vi "HENES.vi"() -> ()   [LabVIEW 2024]
uses:
  <vilib>/Instr/_visa.llb/VISA Set IO Buffer Mask.ctl
  <vilib>/Instr/_visa.llb/VISA Flush IO Buffer Mask.ctl
  <vilib>/Instr/_visa.llb/VISA Configure Serial Port (Instr).vi
panel:
  in  "탭 컨트롤":enum32{"Main"}(tab)
  in  "HLV_A/M":bool=TRUE
  out "Remote_M/A":bool
  out "E-STOP":bool=TRUE
  out "Alive_PCU":u8(slide)=1 scale=0.0..254.0
  out "Speed_Feed(RPM)":dbl format="%#_g rpm"
  in  "HLV_E-stop":bool
  out "Speed_Feed(m/s)":dbl
  in  "InputSteer(cmd)":dbl=28.559259641865033
  out "Steer_Feed":dbl=-0.28
  in  "HLV_Gear":u8
  out "Gear_Feed":u8=1
  out "HENES Loop Time":u32=48
  in  "HENES":refnum<visa-resource-name>="COM3"
  out "버퍼 읽기":string
  out "버퍼 쓰기":string
  in  "InputSpeed":i16
  in  "stop":bool
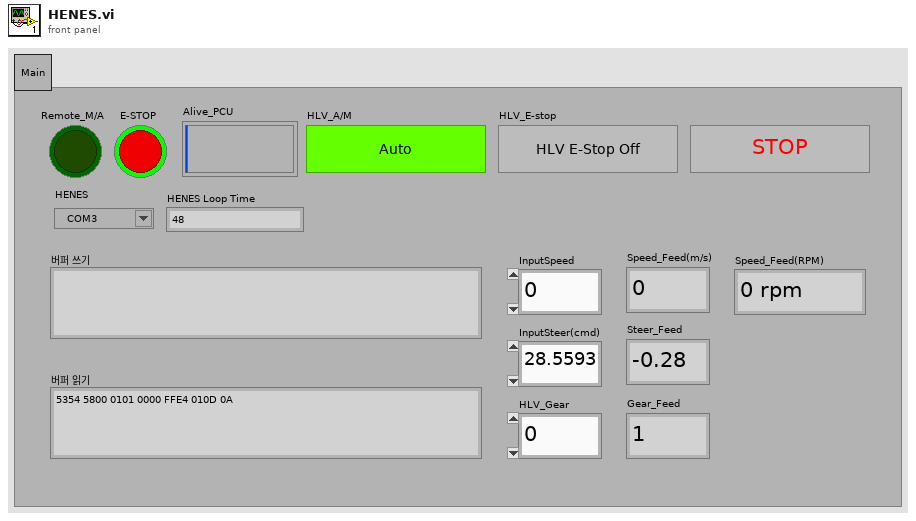
[diagram p1: front panel]
types:
  T1 = cluster{"HENES_M/A":u8, "HENES_E-Stop":u8, "HENES_Gear":u8, "HENES_Speed":i16, "HENES_Steer":i16, "HENES_Alive":u8}
  T2 = typedef "VISA Flush IO Buffer Mask.ctl" = u16
  T3 = typedef "VISA Set IO Buffer Mask.ctl" = u16
  T4 = cluster{"HLV_M/A_Status":u8, "HLV_E-Stop":u8, "HLV_Gear":u8, "HLV_Speed":i16, "HLV_Steer":i16, "HLV_Alive":u8}
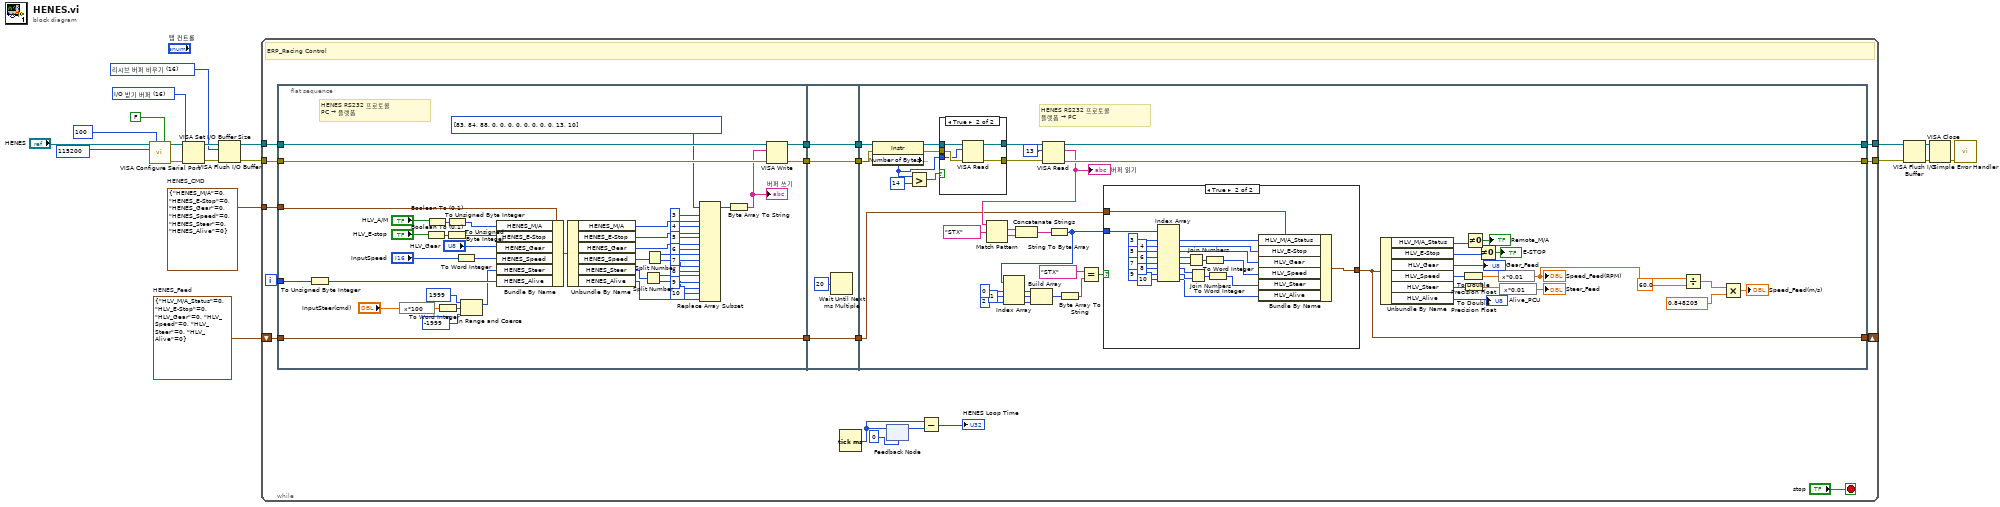
[diagram p0: block diagram]
diagram:
  w2 = T1 {"HENES_M/A"=0, "HENES_E-Stop"=0, "HENES_Gear"=0, "HENES_Speed"=0, "HENES_Steer"=0, "HENES_Alive"=0}  # HENES_CMD
  w5 = T2 16 items=["리시브 버퍼 비우기"=16, "전달 버퍼 디바이스에 쓰기"=32, "리시브 버퍼 비우기(I/O 없음)"=64, "전달 버퍼 비우기"=128] ("Mask")
  w8 = T3 16 items=["I/O 받기 버퍼"=16, "I/O 전달 버퍼"=32, "I/O 받기와 전달 버퍼"=48] ("Mask")
  w12 = T4 {"HLV_M/A_Status"=0, "HLV_E-Stop"=0, "HLV_Gear"=0, "HLV_Speed"=0, "HLV_Steer"=0, "HLV_Alive"=0}  # HENES_Feed
  n1 = call-poly "VISA Configure Serial Port"("VISA resource name"="HENES", "timeout (10sec)"=u32 100, "Enable Termination\nChar (T)"=FALSE ("Enable Termination\nChar (T)"), "baud rate (9600)"=u32 115200) -> ("VISA resource name out"=w4:refnum<visa-resource-name>, "error out"=w3:errorcluster)  [unwired: 10 in]
  n2 = VISA Set I/O Buffer Size(VISA resource name=w4, mask (16)=w8, error in (no error)=w3) -> (VISA resource name out=w7:refnum<visa-resource-name>, error out=w6:errorcluster)  [unwired: 1 in]
  n3 = VISA Flush I/O Buffer(VISA resource name=w7, mask (16)=w5, error in (no error)=w6) -> (VISA resource name out=w17:refnum<visa-resource-name>, error out=w16:errorcluster)
  n4 = while {
    tunnel: w17 -> [w38]
    tunnel: w16 -> [w37]
    tunnel: [w31] -> w15
    tunnel: [w30] -> w14
    shift-right: [w25] -> _
    shift-left: w12 -> [w28]
    tunnel: w2 -> [w26]
    i -> [w32]
    stop <- "stop" stop-if-true
    # "ERP_Racing Control"
    n5 = flat-sequence {
      tunnel: [w81] -> w35
      tunnel: [w80] -> w33
      tunnel: w38 -> [w83]
      tunnel: w37 -> [w82]
      tunnel: w32 -> [w79]
      tunnel: [w78] -> w29
      tunnel: w28 -> [w78]
      tunnel: w26 -> [w77]
      tunnel: [w87] -> w36
      tunnel: w35 -> [w87]
      tunnel: [w86] -> w34
      tunnel: w33 -> [w86]
      tunnel: w29 -> [w84]
      tunnel: [w84] -> w27
      tunnel: w36 -> [w115]
      tunnel: w34 -> [w114]
      tunnel: [w132] -> w31
      tunnel: [w131] -> w30
      tunnel: w27 -> [w106]
      tunnel: [w104] -> w25
      frame #0 {
        # "HENES RS232 프로토콜\nPC → 플랫폼"
        n6 = To Unsigned Byte Integer(number=w79) -> (unsigned 8bit integer=w68:u8)
        n7 = expression code="x*100"("InputSteer(cmd)") -> (w43:dbl)
        n8 = Boolean To (0,1)(Boolean="HLV_E-stop") -> (0, 1=w63:i16)
        n9 = Boolean To (0,1)(Boolean="HLV_A/M") -> (0, 1=w64:i16)
        n10 = To Word Integer(number=w43) -> (16bit integer=w46:i16)
        n11 = To Unsigned Byte Integer(number=w63) -> (unsigned 8bit integer=w61:u8)
        n12 = To Unsigned Byte Integer(number=w64) -> (unsigned 8bit integer=w62:u8)
        n13 = To Word Integer(number="InputSpeed") -> (16bit integer=w55:i16)
        n14 = In Range and Coerce(upper limit=i16 1999 ("상위 리미트"), x=w46, lower limit=i16 -1999 ("상위 리미트")) -> (coerced(x)=w54:i16)  [unwired: 1 out]
        n15 = Bundle By Name(cluster=w77, "HENES_M/A"=w62, "HENES_E-Stop"=w61, "HENES_Gear"="HLV_Gear", "HENES_Speed"=w55, "HENES_Steer"=w54, "HENES_Alive"=w68) -> (w70:T1)
        n16 = Unbundle By Name(w70) -> ("HENES_M/A"=w58:u8, "HENES_E-Stop"=w57:u8, "HENES_Gear"=w47:u8, "HENES_Speed"=w50:i16, "HENES_Steer"=w53:i16, "HENES_Alive"=w67:u8)
        n17 = Split Number(x=w53) -> (hi(x)=w52:u8, lo(x)=w51:u8)
        n18 = Split Number(x=w50) -> (hi(x)=w49:u8, lo(x)=w48:u8)
        n19 = Replace Array Subset(array=u8[] [83, 84, 88, 0, 0, 0, 0, 0, 0, 0, 0, 13, 10] ("unsigned byte array"), new element #1=w58, index #1=3, new element #2=w57, index #2=4, new element #3=w47, index #3=5, new element #4=w49, index #4=6, new element #5=w48, index #5=7, new element #6=w52, index #6=8, new element #7=w51, index #7=9, new element #8=w67, index #8=10) -> (w39:u8[])
        n20 = Byte Array To String(unsigned byte array=w39) -> (string=w41:string)
        "버퍼 쓰기" <- w41
        n21 = VISA Write(VISA resource name=w83, write buffer=w41, error in (no error)=w82) -> (VISA resource name out=w81:refnum<visa-resource-name>, error out=w80:errorcluster)  [unwired: 1 out]
      }
      frame #1 {
        n22 = Wait Until Next ms Multiple(millisecond multiple=u32 20 ("대기 시간 (ms)")) -> ()  [unwired: 1 out]
      }
      frame #2 {
        # "HENES RS232 프로토콜\n플랫폼 → PC"
        n23 = property class="Instr"(reference=w115, error in=w114) -> (reference out=w95:refnum<visa-resource-name>, error out=w94:errorcluster, "Serial Settings:Number of Bytes at Serial Port"=w93:u32)
        n24 = Greater?(x=w93, y=u32 14) -> (0:w111:bool)
        n25 = case shown="True" w111 {
          tunnel: w95 -> [w159 w164]
          tunnel: w94 -> [w158 w163]
          tunnel: [w159 w162] -> w113
          tunnel: [w158 w161] -> w112
          tunnel: w93 -> [_ w160]
          frame False {
          }
          frame True {
            n26 = VISA Read(VISA resource name=w164, byte count=w160, error in (no error)=w163) -> (VISA resource name out=w162:refnum<visa-resource-name>, error out=w161:errorcluster)  [unwired: 2 out]
          }
        }
        n27 = VISA Read(VISA resource name=w113, byte count=u32 13, error in (no error)=w112) -> (VISA resource name out=w132:refnum<visa-resource-name>, read buffer=w130:string, error out=w131:errorcluster)  [unwired: 1 out]
        "버퍼 읽기" <- w130
        n28 = Match Pattern(string=w130, regular expression="STX") -> (match substring=w127:string, after substring=w128:string)  [unwired: 1 in, 2 out]
        n29 = Concatenate Strings(w127, w128) -> (w126:string)
        n30 = String To Byte Array(string=w126) -> (unsigned byte array=w108:u8[])
        n31 = Index Array(array=w108, index #1=0, index #2=1, index #3=2) -> (element #1=w121:u8, element #2=w120:u8, element #3=w119:u8)
        n32 = Build Array(w121, w120, w119) -> (w118:u8[])
        n33 = Byte Array To String(unsigned byte array=w118) -> (string=w116:string)
        n34 = Equal?(x="STX", y=w116) -> (x = y?=w107:bool)
        n35 = case shown="True" w107 {
          tunnel: w108 -> [_ w157]
          tunnel: [w134 w144] -> w104
          tunnel: w106 -> [w134 w146]
          frame False {
          }
          frame True {
            n36 = Index Array(array=w157, index #1=3, index #2=4, index #3=5, index #4=6, index #5=7, index #6=8, index #7=9, index #8=10) -> (element #1=w145:u8, element #2=w143:u8, element #3=w142:u8, element #4=w141:u8, element #5=w140:u8, element #6=w138:u8, element #7=w137:u8, element #8=w135:u8)
            n37 = Join Numbers(hi=w141, lo=w140) -> ((hi.lo)=w148:u16)
            n38 = Join Numbers(hi=w138, lo=w137) -> ((hi.lo)=w147:u16)
            n39 = To Word Integer(number=w148) -> (16bit integer=w139:i16)
            n40 = To Word Integer(number=w147) -> (16bit integer=w136:i16)
            n41 = Bundle By Name(cluster=w146, "HLV_M/A_Status"=w145, "HLV_E-Stop"=w143, "HLV_Gear"=w142, "HLV_Speed"=w139, "HLV_Steer"=w136, "HLV_Alive"=w135) -> (w144:T4)
          }
        }
        n42 = Unbundle By Name(w104) -> ("HLV_M/A_Status"=w105:u8, "HLV_E-Stop"=w99:u8, "HLV_Gear"=→"Gear_Feed":u8, "HLV_Speed"=w97:i16, "HLV_Steer"=w96:i16, "HLV_Alive"=→"Alive_PCU":u8)
        n43 = To Double Precision Float(number=w97) -> (double precision float=w109:dbl)
        n44 = To Double Precision Float(number=w96) -> (double precision float=w102:dbl)
        n45 = Not Equal To 0?(x=w105) -> (x != 0?=→"Remote_M/A":bool)
        n46 = Not Equal To 0?(x=w99) -> (x != 0?=→"E-STOP":bool)
        n47 = expression code="x*0.01"(w109) -> (w88:dbl)
        "Speed_Feed(RPM)" <- w88
        n48 = expression code="x*0.01"(w102) -> (→"Steer_Feed":dbl)
        n49 = Divide(x=w88, y=60.0) -> (x/y=w92:dbl)
        n50 = Multiply(x=w92, y=0.848205) -> (x*y=→"Speed_Feed(m/s)":dbl)
      }
    }
    n51 = Tick Count (ms)() -> (millisecond timer value=w22:u32)
    n52 = feedback #1(u32 0 ("millisecond timer value")) -> (w23:u32)
    n53 = feedback-in #1(w22) -> ()
    n54 = Subtract(x=w22, y=w23) -> (x-y=→"HENES Loop Time":u32)
  }
  n55 = VISA Flush I/O Buffer(VISA resource name=w15, error in (no error)=w14) -> (VISA resource name out=w18:refnum<visa-resource-name>, error out=w19:errorcluster)  [unwired: 1 in]
  n56 = VISA Close(VISA resource name=w18, error in (no error)=w19) -> (error out=w13:errorcluster)
  n57 = call <vilib>:"Simple Error Handler.vi"("error in (no error)"=w13) -> ()  [unwired: 4 in, 5 out]
